vi "Configure Programmer Parameters (Program Hold).vi"(0 "VISA resource name":refnum<visa-resource-name>, 1 "Unit Address (1)":u8=1, 2 "Number of Cycles Remaining (0)":i16 min=-1 max=1000, 5 "Programmer Setpoint (0)":i16, 7 "Segment Time Remaining (0)":i16, 9 "Current Target Setpoint Value (0)":i16, 11 "error in (no error)":errorcluster, 12 "Segment Ramp Rate (1)":u16=1 min=1, 13 "Event Outputs (0)":bool[](array[boolean])) -> (4 "VISA resource name out":refnum<visa-resource-name>, 15 "error out":errorcluster)   [LabVIEW 2014, in "Eurotherm 35xx Series.lvlib"]
doc: "This VI sets Output Parameters."
uses:
  <instrlib>/Eurotherm 35xx Series/Eurotherm 35xx Series.lvlib
panel:
  # "1"
  # "2"
  # "3"
  # "4"
  # "5"
  # "6"
  # "7"
  # "8"
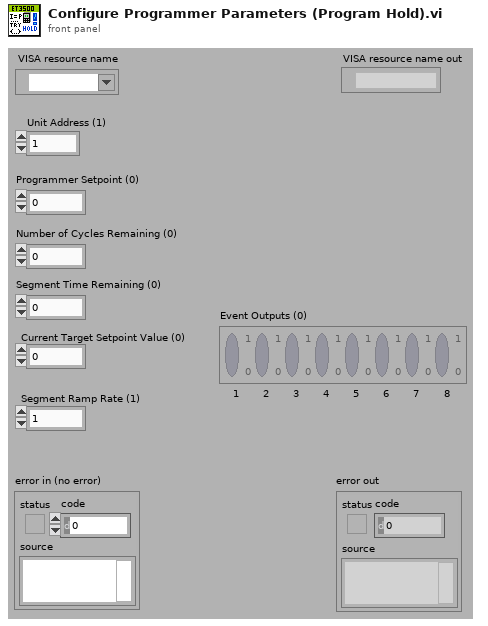
[diagram p1: front panel]
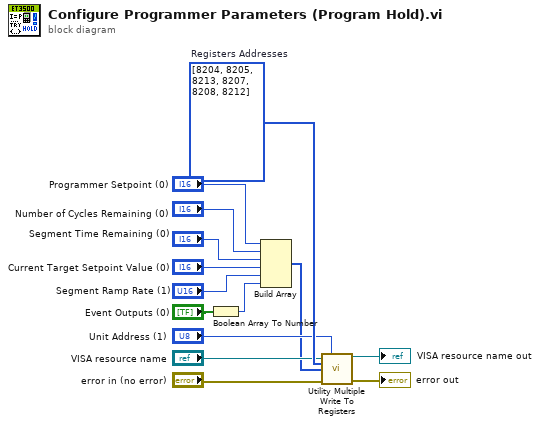
[diagram p0: block diagram]
diagram:
  w12 = u16[] [8204, 8205, 8213, 8207, 8208, 8212]  # Registers Addresses
  n1 = Boolean Array To Number(Boolean array="Event Outputs (0)") -> (number=w7:u32)
  n2 = Build Array("Programmer Setpoint (0)", "Number of Cycles Remaining (0)", "Segment Time Remaining (0)", "Current Target Setpoint Value (0)", "Segment Ramp Rate (1)", w7) -> (w1:u32[])
  n3 = call <instrlib>:"Utility Multiple Write To Registers.vi"("VISA resource name"="VISA resource name", "Unit Address (1)"="Unit Address (1)", "Registers Addresses (0)"=w12, "Data (0)"=w1, "error in (no error)"="error in (no error)") -> ("VISA resource name out"=→"VISA resource name out":refnum<visa-resource-name>, "error out"=→"error out":errorcluster)  [unwired: 9 in]
